vi "CRYPEAQ Makeing TSR FlFcFu.vi"(7 "Sweep time":dbl=1.0 format="%.2f", 8 "Fstop":dbl=20000.0 format="%.2f", 9 "Fstart":dbl=20.0 format="%.2f", 10 "Fs":dbl=44100.0 format="%.2f") -> (0 "Fu Index":i32[](array[numeric]), 1 "Fu":dbl[](array[numeric])=[22.454773997922736, 22.97758714371529, 23.51258021383542, 24.060036879710538, 24.6202474215474, 25.193508881725744, 25.780125222574476, 26.380407487261397, 26.99467396487717, 27.62325035931701, 28.26646996176788, 28.92467382730014, 29.598210956047147, 30.287438477900952, 30.992721842290486, 31.714435011380765, 32.452960658853264, 33.208690372401655, 33.98202486161858, 34.773374170387285, 35.58315789437015, 36.41180540330013, 37.259756068478765, 38.127459496456304, 39.01537576663182, 39.923975675444694, 40.85374098616558, 41.80516468428786, 42.77875123862532, 43.77501686920085, 44.79448982064225, 45.83771064227755, 46.90523247502523, 47.99762134429284, 49.115456460467634, 50.2593305257138, 51.42985004836605, 52.62763566442533, 53.85332246665549, 55.10756034167334, 56.391014313751576, 57.70436489820836, 59.04830846170678, 60.423557591748676, 61.830841474273164, 63.27090628064966, 64.74451556287737, 66.25245065877897, 67.79551110590032, 69.37451506590403, 70.9902997579681, 72.64372190278358, 74.33565817714842, 76.0670056781684, 77.83868239945207, 79.65162771770717, 81.50680289034209, 83.40519156605784, 85.34780030545036, 87.33565911540498, 89.36982199479563, 91.45136749348208, 93.58139928410841, 95.76104674749965, 97.99146557116102, 100.27383836227469, 102.60937527440015, 104.99931464986868, 107.44492367538494, 109.94749905452376, 112.5083676952281, 115.12888741310817, 117.8104476515396, 120.55447021846123, 123.36241003987485, 126.23575593174236, 129.1760313889854, 132.18479539348297, 135.26364324037172, 138.4142073845422, 141.63815830533997, 144.93720539296265, 148.31309785436, 151.76762564113122, 155.30262039792564, 158.91995643433984, 162.62155171801825, 166.4093688923503, 170.2854163162711, 174.251749129759, 178.31047034303583, 182.46373195196514, 186.71373607895154, 191.06273614043988, 195.51303804181413, 200.06700139989707, 204.72704079434857, 209.49562704746577, 214.37528853468135, 219.3686125246637, 224.47824655161554, 229.70689981887307, 235.057344635006, 240.53241788431615, 246.135022530637, 251.86812915653312, 257.73477753839944, 263.73807825806085, 269.881214352571, 276.1674430011124, 282.6000972524956, 289.18258779245804, 295.91840475156465, 302.81111955630627, 309.8643868222997, 317.081946292187, 324.4676248185348, 332.0253383927343, 339.75909422140023, 347.67299285107083, 355.7712303422073, 364.0581004944929, 372.5379971226333, 381.2154163868554, 390.0949591762076, 399.1813335484587, 408.47935722609816, 417.99396015083505, 427.7301870974983, 437.6932003488361, 447.8882824328153, 458.3208389232213, 468.99640130595765, 479.92062991154586, 491.09931691702474, 502.5383894162503, 514.2439125630955, 526.2220927869496, 538.4792810835186, 551.0219763824239, 563.8568289927026, 576.9906441289077, 590.4303855198066, 604.1831790999819, 618.2563167885307, 632.6572603549645, 647.3936453762086, 662.4732852843022, 677.9041755094981, 693.6944977199626, 709.8526241591744, 726.387122085026, 743.3067583130218, 760.6205038636788, 778.3375387195264, 796.4672566926057, 815.0192704046698, 834.0034163843833, 853.429760282622, 873.3086022095733, 893.6504821954353, 914.4661857797167, 935.7667497292374, 957.5634678900275, 979.8678971760271, 1002.6918636957867, 1026.0474690237668, 1049.9470966162373, 1074.4034183769784, 1099.429401376779, 1125.0383147279376, 1151.2437366204622, 1178.059561520769, 1205.5000075390842, 1233.5796239681415, 1262.3132989970838, 1291.716267605563, 1321.8041196417378, 1352.592808087576, 1384.0986575181541, 1416.3383727566554, 1449.329047731571, 1483.0881745401007, 1517.6336527227509, 1552.983798754135, 1589.1573557540758, 1626.173503426001, 1664.0518682259462, 1702.8125337688543, 1742.4760514771751, 1783.0634514774647, 1824.596253750986, 1867.0964795436084, 1910.5866630422083, 1955.0898633219676, 2000.629676573275, 2047.2302486121253, 2094.916287683119, 2143.7130775595638, 2193.6464909496717, 2244.7430032145617, 2297.0297064054575, 2350.534323628789, 2405.2852237450925, 2461.3114364103076, 2518.642667468382, 2577.309314700866, 2637.342483944817, 2698.774005585298, 2761.636451432274, 2825.9631519907193, 2891.788214132709, 2959.1465391814268, 3028.073841416658, 3098.6066670100945, 3170.7824134035327, 3244.6393491370727, 3320.21663413942, 3397.554340491384, 3476.69347367248, 3557.675994302525, 3640.544840389543, 3725.3439500966592, 3812.118285038006, 3900.9138541182183, 3991.777737927235, 4084.7581137026004, 4179.904280874161, 4277.266687202766, 4376.896955528673, 4478.84791114254, 4583.173609794229, 4689.9293663536055, 4799.17178413954, 4910.958784931605, 5025.349639680679, 5142.40499993584, 5262.186930001873, 5384.7589398471655, 5510.186018777306, 5638.534669893191, 5769.872945352114, 5904.270482449578, 6041.798540542085, 6182.530038829943, 6326.539595019659, 6473.903564887547, 6624.700082764322, 6779.009102963305, 6936.912442172715, 7098.493822836377, 7263.838917544618, 7433.0353944582685, 7606.172963792461, 7783.34342538143, 7964.640717352117, 8150.16096593186, 8340.002536415303, 8534.266085318994, 8733.05461375138, 8936.473522024511, 9144.630665539245, 9357.636411971636, 9575.60369979094, 9798.648098141424, 18000.0] format="%#.6g", 2 "Fc":dbl[](array[numeric]), 3 "Fl":dbl[](array[numeric])=[20.0, 22.454773997922736, 22.97758714371529, 23.51258021383542, 24.060036879710538, 24.6202474215474, 25.193508881725744, 25.780125222574476, 26.380407487261397, 26.99467396487717, 27.62325035931701, 28.26646996176788, 28.92467382730014, 29.598210956047147, 30.287438477900952, 30.992721842290486, 31.714435011380765, 32.452960658853264, 33.208690372401655, 33.98202486161858, 34.773374170387285, 35.58315789437015, 36.41180540330013, 37.259756068478765, 38.127459496456304, 39.01537576663182, 39.923975675444694, 40.85374098616558, 41.80516468428786, 42.77875123862532, 43.77501686920085, 44.79448982064225, 45.83771064227755, 46.90523247502523, 47.99762134429284, 49.115456460467634, 50.2593305257138, 51.42985004836605, 52.62763566442533, 53.85332246665549, 55.10756034167334, 56.391014313751576, 57.70436489820836, 59.04830846170678, 60.423557591748676, 61.830841474273164, 63.27090628064966, 64.74451556287737, 66.25245065877897, 67.79551110590032, 69.37451506590403, 70.9902997579681, 72.64372190278358, 74.33565817714842, 76.0670056781684, 77.83868239945207, 79.65162771770717, 81.50680289034209, 83.40519156605784, 85.34780030545036, 87.33565911540498, 89.36982199479563, 91.45136749348208, 93.58139928410841, 95.76104674749965, 97.99146557116102, 100.27383836227469, 102.60937527440015, 104.99931464986868, 107.44492367538494, 109.94749905452376, 112.5083676952281, 115.12888741310817, 117.8104476515396, 120.55447021846123, 123.36241003987485, 126.23575593174236, 129.1760313889854, 132.18479539348297, 135.26364324037172, 138.4142073845422, 141.63815830533997, 144.93720539296265, 148.31309785436, 151.76762564113122, 155.30262039792564, 158.91995643433984, 162.62155171801825, 166.4093688923503, 170.2854163162711, 174.251749129759, 178.31047034303583, 182.46373195196514, 186.71373607895154, 191.06273614043988, 195.51303804181413, 200.06700139989707, 204.72704079434857, 209.49562704746577, 214.37528853468135, 219.3686125246637, 224.47824655161554, 229.70689981887307, 235.057344635006, 240.53241788431615, 246.135022530637, 251.86812915653312, 257.73477753839944, 263.73807825806085, 269.881214352571, 276.1674430011124, 282.6000972524956, 289.18258779245804, 295.91840475156465, 302.81111955630627, 309.8643868222997, 317.081946292187, 324.4676248185348, 332.0253383927343, 339.75909422140023, 347.67299285107083, 355.7712303422073, 364.0581004944929, 372.5379971226333, 381.2154163868554, 390.0949591762076, 399.1813335484587, 408.47935722609816, 417.99396015083505, 427.7301870974983, 437.6932003488361, 447.8882824328153, 458.3208389232213, 468.99640130595765, 479.92062991154586, 491.09931691702474, 502.5383894162503, 514.2439125630955, 526.2220927869496, 538.4792810835186, 551.0219763824239, 563.8568289927026, 576.9906441289077, 590.4303855198066, 604.1831790999819, 618.2563167885307, 632.6572603549645, 647.3936453762086, 662.4732852843022, 677.9041755094981, 693.6944977199626, 709.8526241591744, 726.387122085026, 743.3067583130218, 760.6205038636788, 778.3375387195264, 796.4672566926057, 815.0192704046698, 834.0034163843833, 853.429760282622, 873.3086022095733, 893.6504821954353, 914.4661857797167, 935.7667497292374, 957.5634678900275, 979.8678971760271, 1002.6918636957867, 1026.0474690237668, 1049.9470966162373, 1074.4034183769784, 1099.429401376779, 1125.0383147279376, 1151.2437366204622, 1178.059561520769, 1205.5000075390842, 1233.5796239681415, 1262.3132989970838, 1291.716267605563, 1321.8041196417378, 1352.592808087576, 1384.0986575181541, 1416.3383727566554, 1449.329047731571, 1483.0881745401007, 1517.6336527227509, 1552.983798754135, 1589.1573557540758, 1626.173503426001, 1664.0518682259462, 1702.8125337688543, 1742.4760514771751, 1783.0634514774647, 1824.596253750986, 1867.0964795436084, 1910.5866630422083, 1955.0898633219676, 2000.629676573275, 2047.2302486121253, 2094.916287683119, 2143.7130775595638, 2193.6464909496717, 2244.7430032145617, 2297.0297064054575, 2350.534323628789, 2405.2852237450925, 2461.3114364103076, 2518.642667468382, 2577.309314700866, 2637.342483944817, 2698.774005585298, 2761.636451432274, 2825.9631519907193, 2891.788214132709, 2959.1465391814268, 3028.073841416658, 3098.6066670100945, 3170.7824134035327, 3244.6393491370727, 3320.21663413942, 3397.554340491384, 3476.69347367248, 3557.675994302525, 3640.544840389543, 3725.3439500966592, 3812.118285038006, 3900.9138541182183, 3991.777737927235, 4084.7581137026004, 4179.904280874161, 4277.266687202766, 4376.896955528673, 4478.84791114254, 4583.173609794229, 4689.9293663536055, 4799.17178413954, 4910.958784931605, 5025.349639680679, 5142.40499993584, 5262.186930001873, 5384.7589398471655, 5510.186018777306, 5638.534669893191, 5769.872945352114, 5904.270482449578, 6041.798540542085, 6182.530038829943, 6326.539595019659, 6473.903564887547, 6624.700082764322, 6779.009102963305, 6936.912442172715, 7098.493822836377, 7263.838917544618, 7433.0353944582685, 7606.172963792461, 7783.34342538143, 7964.640717352117, 8150.16096593186, 8340.002536415303, 8534.266085318994, 8733.05461375138, 8936.473522024511, 9144.630665539245, 9357.636411971636, 9575.60369979094, 9798.648098141424] format="%#.6g")   [LabVIEW 2013]
panel:
  out "Waveform Graph 6":i32[](graph)
  out "max value":i32
  out "Waveform Graph 5":i32[](graph)
  out "Center Frequency Index":i32[](array[numeric])
  out "All Frequency":dbl[](array[numeric])
  out "Frequecy Array":i32
  out "All Samples":i32
  out "Waveform Graph 3":dbl[](graph)
  out "All Time":dbl
  out "Waveform Graph 2":dbl[](graph)
  out "size(s) 3":i32
  out "Waveform Graph":waveform(dbl)(graph)
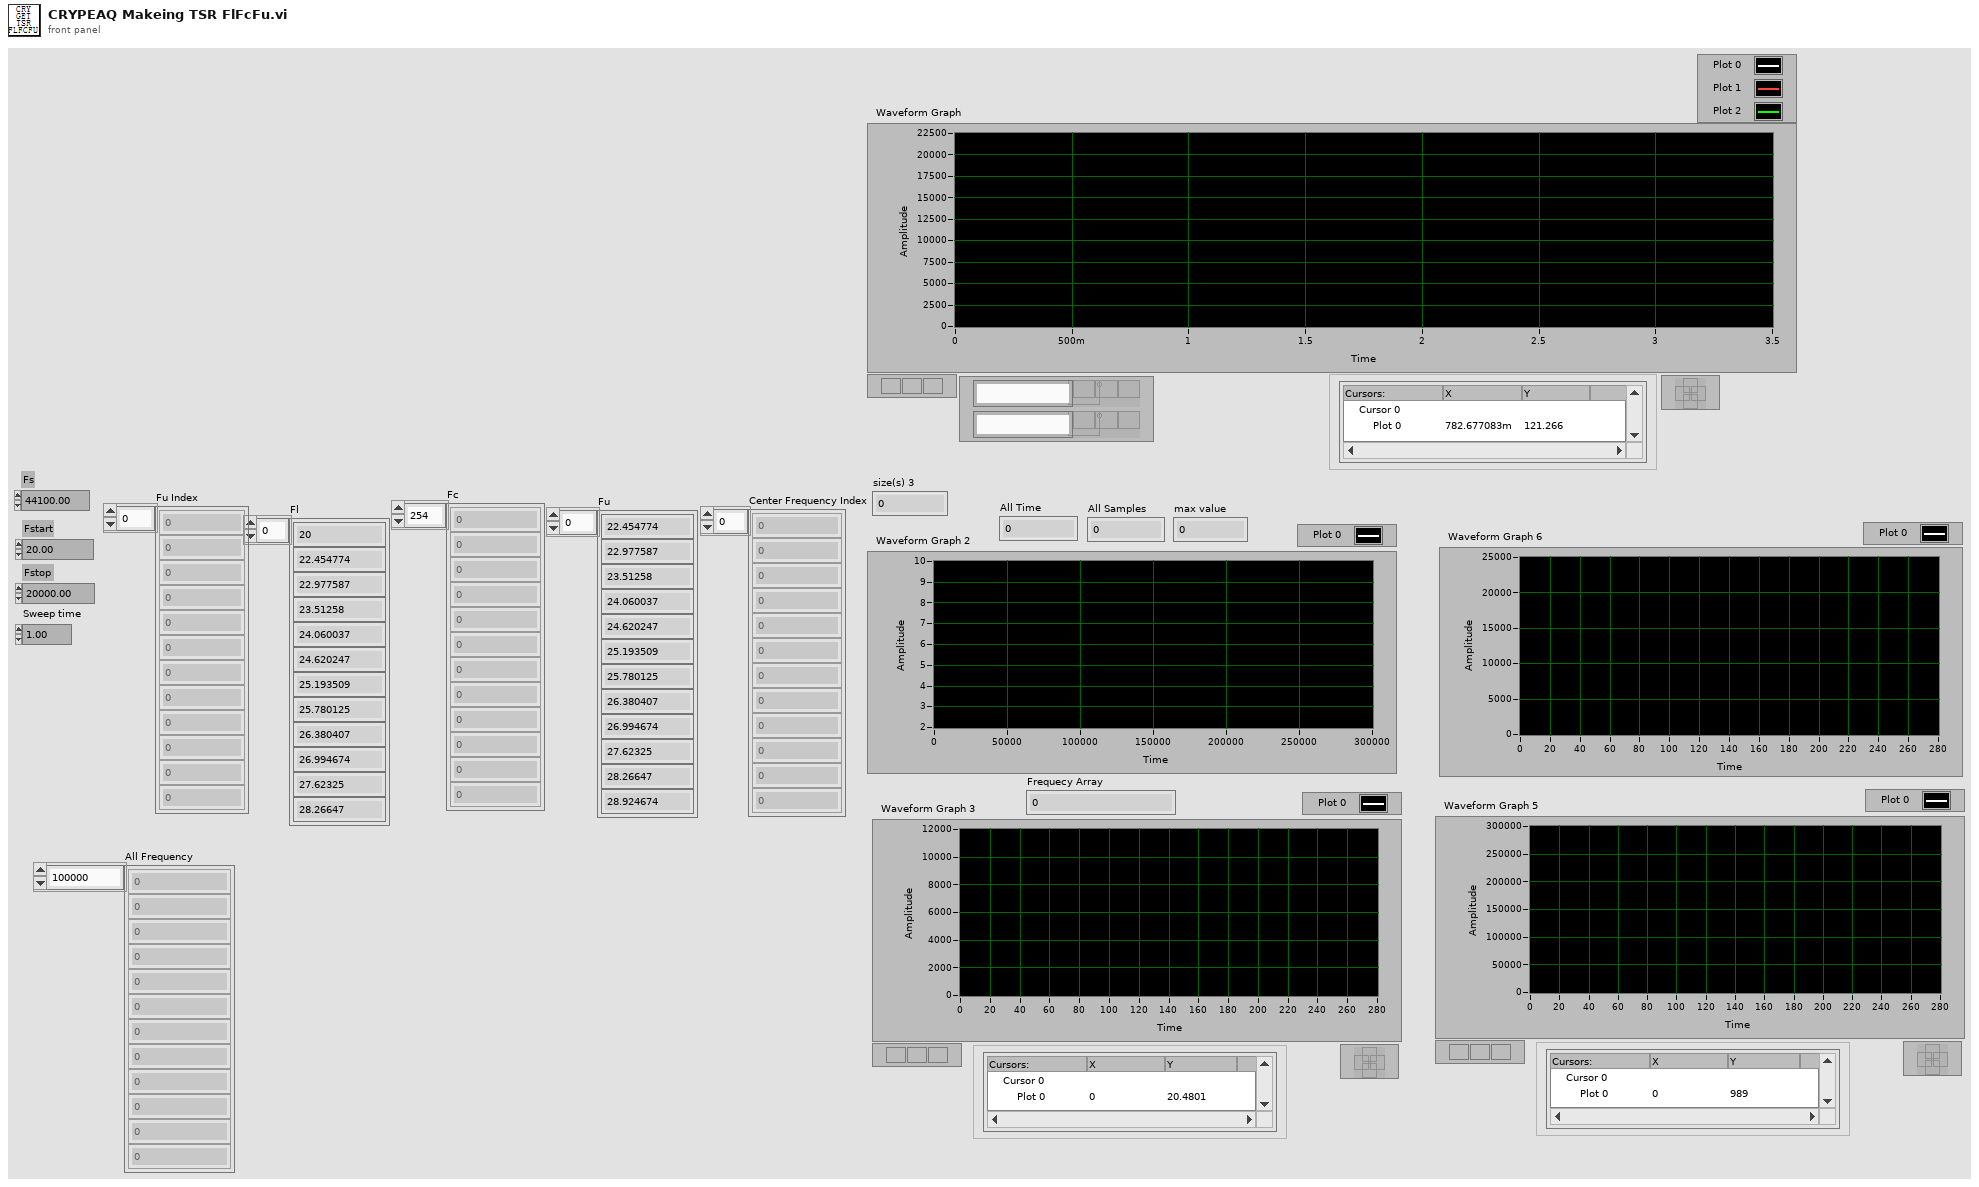
[diagram p1: front panel]
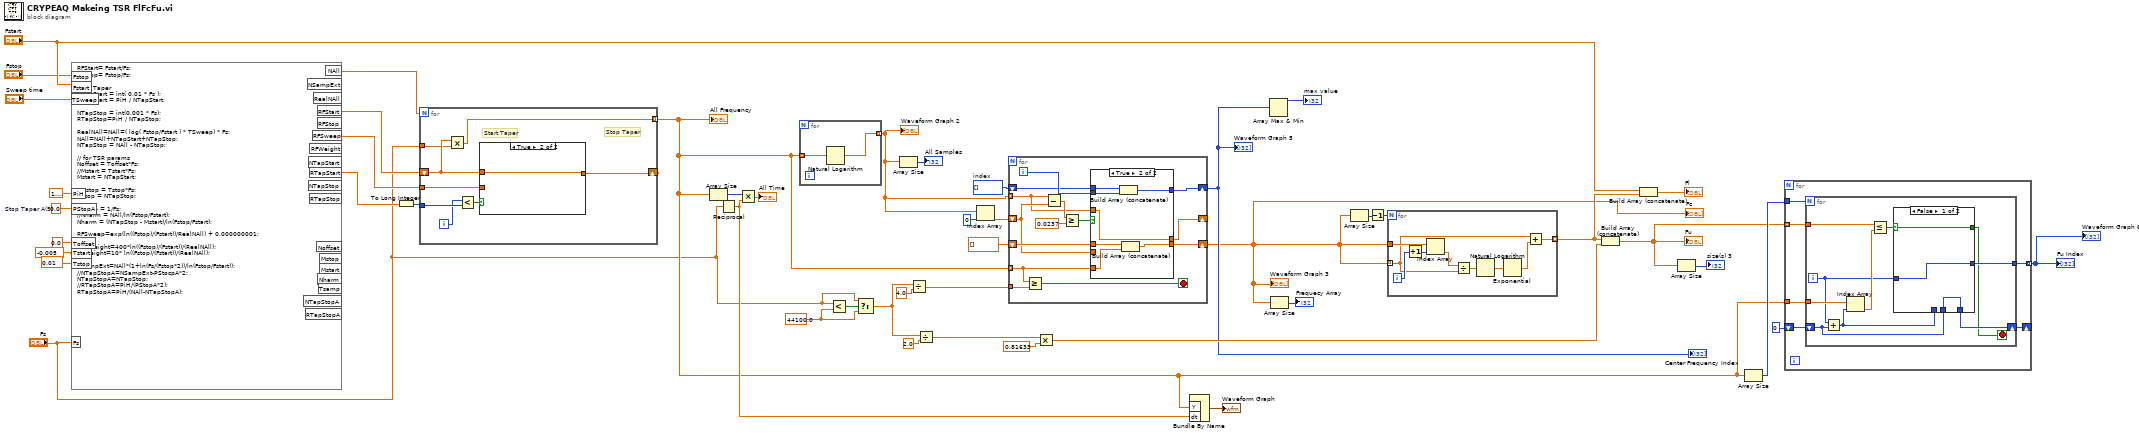
[diagram p0: block diagram]
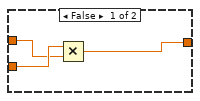
[diagram p3: hidden frame]
diagram:
  w2 = 44100.0 ("Fs")
  w21 = i32[] []  # index
  w41 = 0.0  # Stop Taper A(5)
  n1 = formula code="RFStart= Fstart/Fs;\nRFStop= Fstop/Fs;\n\n// for Taper\nNTapStart = int( 0.01 * Fs );\nRTapStart = PiH / NTapStart;\n\nNTapStop = int(0.001 * Fs);\nRTapStop=PiH / NTapStop;\n\nRealNAll=NAll=( log( Fstop/Fstart ) * TSweep) * Fs;\nNAll=NAll+NTapStart+NTapStop;\nNTapStop = NAll - NTapStop;\n\n// for TSR params\nNoffset = Toffset*Fs;\n//Mstart = Tstart*Fs;\nMstart = NTapStart;\n\n//Mstop = Tstop*Fs;\nMstop = NTapStop;\n\nTsamp = 1/Fs;\n//Nharm = NAll/ln(Fstop/Fstart);\nNharm = (NTapStop - Mstart)/ln(Fstop/Fstart); \n\nRFSweep=exp(ln((Fstop)/(Fstart))/RealNAll) + 0.000000001;\n\n//RFWeight=400*ln((Fstop)/(Fstart))/(RealNAll);\nRFWeight=10* ln((Fstop)/(Fstart))/(RealNAll);\n\nNSampExt=NAll*(1+ln(Fs/(Fstop*2))/ln(Fstop/Fstart));\n//NTapStopA=NSampExt-PStocpA*2;\nNTapStopA=NTapStop;\n//RTapStopA=PiH/(PStopA*2);\nRTapStopA=PiH/(NAll-NTapStopA);"("TSweep"="Sweep time", "Fstop"="Fstop", "Fstart"="Fstart", "Fs"="Fs", "PiH"=1.5707963267948966, "PStopA"=w41, "Tstart"=-0.005, "Tstop"=0.01, "Toffset"=0.0) -> ("RFStart"=w25:dbl, "RFSweep"=w26:dbl, "RTapStart"=w24:dbl, "NAll"=w22:dbl)  [unwired: 14 out]
  n2 = To Long Integer(number=w24) -> (32bit integer=w23:i32)
  n3 = for {
    N: w22 -> [_]
    tunnel: w23 -> [w54]
    tunnel: w26 -> [w52]
    shift-right: [w51] -> _
    shift-left: w25 -> [w50]
    tunnel: [w48] -> w5 mode=indexing
    tunnel: "Fs" -> [w49]
    i -> [w53]
    # "Start Taper"
    # "Stop Taper"
    n4 = Multiply(x=w50, y=w49) -> (x*y=w48:dbl)
    n5 = Less?(x=w53, y=w54) -> (x < y?=w55:bool)
    n6 = case shown="True" w55 {
      tunnel: w52 -> [w57 _]
      tunnel: w50 -> [w56 w59]
      tunnel: [w58 w59] -> w51
      frame False {
        n7 = Multiply(x=w57, y=w56) -> (x*y=w58:dbl)
      }
      frame True {
      }
    }
  }
  "All Frequency" <- w5
  n8 = Array Size(array=w5) -> (size(s)=w36:i32)
  n9 = Reciprocal(x="Fs") -> (1/x=w9:dbl)
  n10 = Multiply(x=w36, y=w9) -> (x*y=→"All Time":dbl)
  n11 = for {
    tunnel: w5 -> [w61] mode=indexing
    tunnel: [w60] -> w30 mode=indexing
    n12 = Natural Logarithm(1:w61) -> (0:w60:dbl)
  }
  "Waveform Graph 2" <- w30
  n13 = Less?(x="Fs", y=w2) -> (x < y?=w4:bool)
  n14 = Select(t="Fs", s=w4, f=w2) -> (s? t:f=w1:dbl)
  n15 = Array Size(array=w30) -> (size(s)=→"All Samples":i32)
  n16 = Divide(x=w1, y=4.0) -> (x/y=w27:dbl)
  n17 = Divide(x=w1, y=2.0) -> (x/y=w15:dbl)
  n18 = Index Array(array=w30, index=0) -> (element=w29:dbl)
  n19 = for {
    tunnel: w30 -> [w65] mode=indexing
    shift-right: [w71] -> _
    shift-left: w29 -> [w69]
    shift-right: [w73] -> w7
    shift-left: dbl[] [] -> [w72]
    tunnel: w5 -> [w68] mode=indexing
    tunnel: w27 -> [w67]
    shift-right: [w63] -> w14
    shift-left: w21 -> [w62]
    i -> [w64]
    stop <- w66 stop-if-true
    n20 = Greater Or Equal?(x=w68, y=w67) -> (x >= y?=w66:bool)
    n21 = Subtract(x=w65, y=w69) -> (x-y=w70:dbl)
    n22 = Greater Or Equal?(x=w70, y=0.0237) -> (x >= y?=w75:bool)
    n23 = case shown="True" w75 {
      tunnel: w69 -> [w77 _]
      tunnel: [w78 w85] -> w73
      tunnel: w72 -> [w78 w84]
      tunnel: [w77 w82] -> w71
      tunnel: w68 -> [_ w83]
      tunnel: w65 -> [_ w82]
      tunnel: w64 -> [_ w81]
      tunnel: [w76 w80] -> w63
      tunnel: w62 -> [w76 w79]
      frame False {
      }
      frame True {
        n24 = Build Array (concatenate)(w79, w81) -> (w80:i32[])
        n25 = Build Array (concatenate)(w84, w83) -> (w85:dbl[])
      }
    }
  }
  "Waveform Graph 3" <- w7
  "Fc" <- w7
  "Center Frequency Index" <- w14
  "Waveform Graph 5" <- w14
  n26 = Multiply(x=w15, y=0.81633) -> (x*y=w16:dbl)
  n27 = Bundle By Name("Y"=w5, "dt"=w9) -> (→"Waveform Graph":waveform(dbl))  [unwired: 1 in]
  n28 = Array Max & Min(array=w14) -> (max value=→"max value":i32)  [unwired: 3 out]
  n29 = Array Size(array=w7) -> (size(s)=→"Frequecy Array":i32)
  n30 = Array Size(array=w7) -> (size(s)=w47:i32)
  n31 = Decrement(x=w47) -> (x-1=w46:i32)
  n32 = for {
    N: w46 -> [_]
    tunnel: w7 -> [w88] mode=indexing
    tunnel: w7 -> [w94]
    tunnel: [w91] -> w44 mode=indexing
    i -> [w93]
    n33 = Increment(x=w93) -> (x+1=w92:i32)
    n34 = Index Array(array=w94, index=w92) -> (element=w87:dbl)
    n35 = Divide(x=w87, y=w88) -> (x/y=w89:dbl)
    n36 = Natural Logarithm(1:w89) -> (0:w86:dbl)
    n37 = Exponential(1:w86) -> (0:w90:dbl)
    n38 = Add(x=w88, y=w90) -> (x+y=w91:dbl)
  }
  n39 = Build Array (concatenate)(w44, w16) -> (w8:dbl[])
  "Fu" <- w8
  n40 = Build Array (concatenate)("Fstart", w44) -> (→"Fl":dbl[])
  n41 = Array Size(array=w8) -> (size(s)=→"size(s) 3":i32)
  n42 = Array Size(array=w5) -> (size(s)=w10:i32)
  n43 = for {
    tunnel: w8 -> [w99] mode=indexing
    tunnel: w5 -> [w100]
    tunnel: [w98] -> w12 mode=indexing
    shift-right: [w96] -> _
    shift-left: 0 -> [w97]
    tunnel: w10 -> [w95]
    n44 = for {
      N: w95 -> [_]
      tunnel: w100 -> [w109]
      tunnel: w99 -> [w108]
      tunnel: [w110] -> w98
      shift-right: [w104] -> w96
      shift-left: w97 -> [w105]
      i -> [w106]
      stop <- w101 stop-if-true
      n45 = Add(x=w106, y=w105) -> (x+y=w103:i32)
      n46 = Index Array(array=w109, index=w103) -> (element=w107:dbl)
      n47 = Less Or Equal?(x=w108, y=w107) -> (x <= y?=w102:bool)
      n48 = case shown="False" w102 {
        selector: w102 -> [w111 w114]
        tunnel: [w112 w116] -> w110
        tunnel: w106 -> [w112 w116]
        tunnel: w105 -> [w113 _]
        tunnel: [w113 w115] -> w104
        tunnel: w103 -> [_ w115]
        tunnel: [w111 w114] -> w101
        frame False {
        }
        frame True {
        }
      }
    }
  }
  "Fu Index" <- w12
  "Waveform Graph 6" <- w12
